vi "drive forward (1).vi"(8 "error in (no error)":errorcluster, 9 "forward":bool=TRUE, 10 "desired distance":dbl, 11 "RobotDriveDevRef in":T1) -> (0 "error out":errorcluster, 3 "RobotDriveDevRef out":T1)   [LabVIEW 2016]
uses:
  <vilib>/Rock Robotics/WPI/RobotDrive/WPI_RobotDriveDevRef.ctl
  <vilib>/Rock Robotics/WPI/MotorControl/WPI_MotorControlDeviceRef.ctl
  <vilib>/Rock Robotics/WPI/MotorControl/WPI_MotorControlType.ctl
  <vilib>/Rock Robotics/SystemInterfaces/DIO/FPGA_DIOPWMChannel.ctl
  <vilib>/Rock Robotics/WPI/PWM/WPI_PWMDeadband.ctl
  <vilib>/Rock Robotics/Network Tables/NT Write Number.vi
  <vilib>/Rock Robotics/WPI/RobotDrive/WPI_RobotDriveArcadeDrive_Standard(NoSaturation).vi
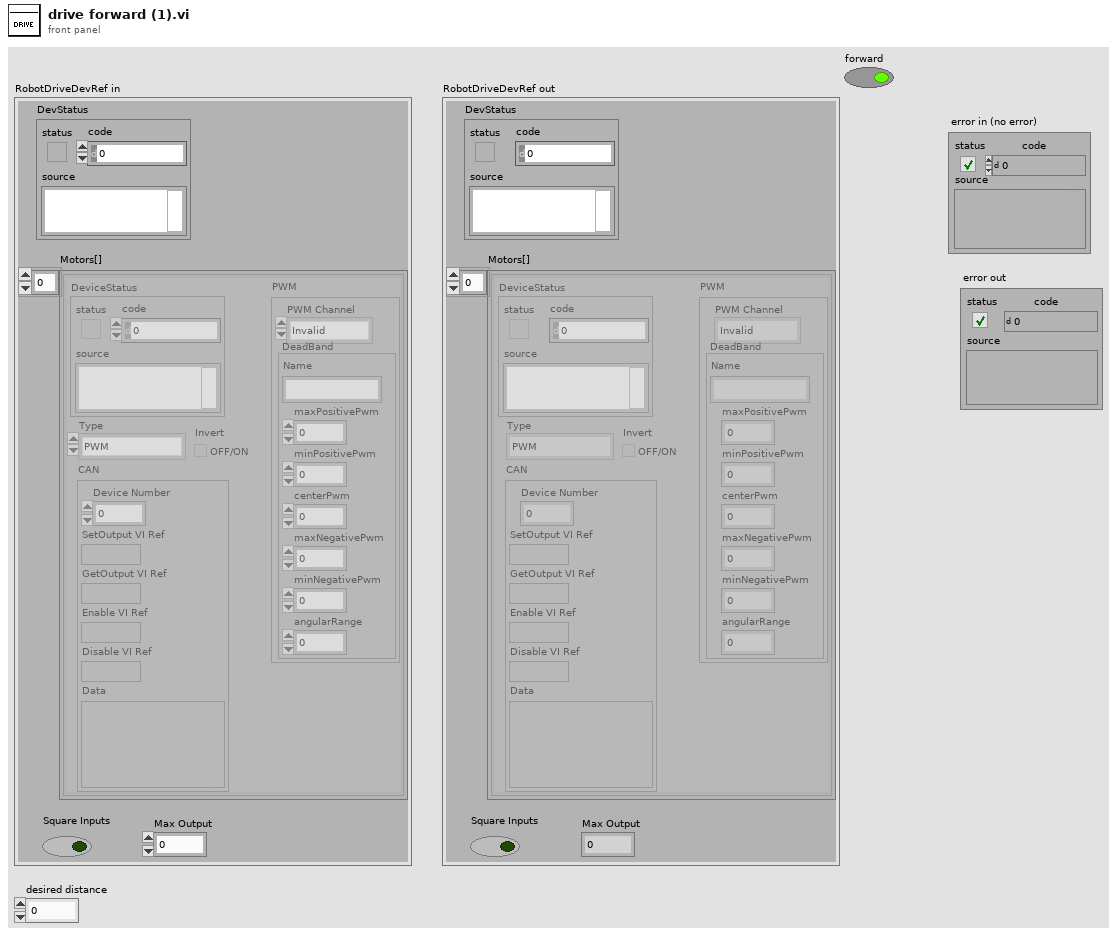
[diagram p1: front panel]
types:
  T1 = typedef "WPI_RobotDriveDevRef.ctl" = cluster{"DevStatus":errorcluster, "Motors[]":T2[], "Square Inputs":bool, "Max Output":dbl}
  T2 = typedef "WPI_MotorControlDeviceRef.ctl" = cluster{"DeviceStatus":errorcluster, "Type":T3, "PWM":cluster{"PWM Channel":T4, "DeadBand":T5}, "CAN":cluster{"Device Number":u8, "SetOutput VI Ref":variant, "GetOutput VI Ref":variant, "Enable VI Ref":variant, "Disable VI Ref":variant, "Data":variant}, "Invert":bool}
  T3 = typedef "WPI_MotorControlType.ctl" = enum16{"PWM", "CAN"}
  T4 = typedef "FPGA_DIOPWMChannel.ctl" = enum8{"PWM 0", "PWM 1", "PWM 2", "PWM 3", "PWM 4", "PWM 5", "PWM 6", "PWM 7", "PWM 8", "PWM 9", "PWM MXP 0", "PWM MXP 1", "PWM MXP 2", "PWM MXP 3", "PWM MXP 4", "PWM MXP 5", "PWM MXP 6", "PWM MXP 7", "PWM MXP 8", "PWM MXP 9", "Invalid"}
  T5 = typedef "WPI_PWMDeadband.ctl" = cluster{"Name":string, "maxPositivePwm":i32, "minPositivePwm":i32, "centerPwm":i32, "maxNegativePwm":i32, "minNegativePwm":i32, "angularRange":u16}
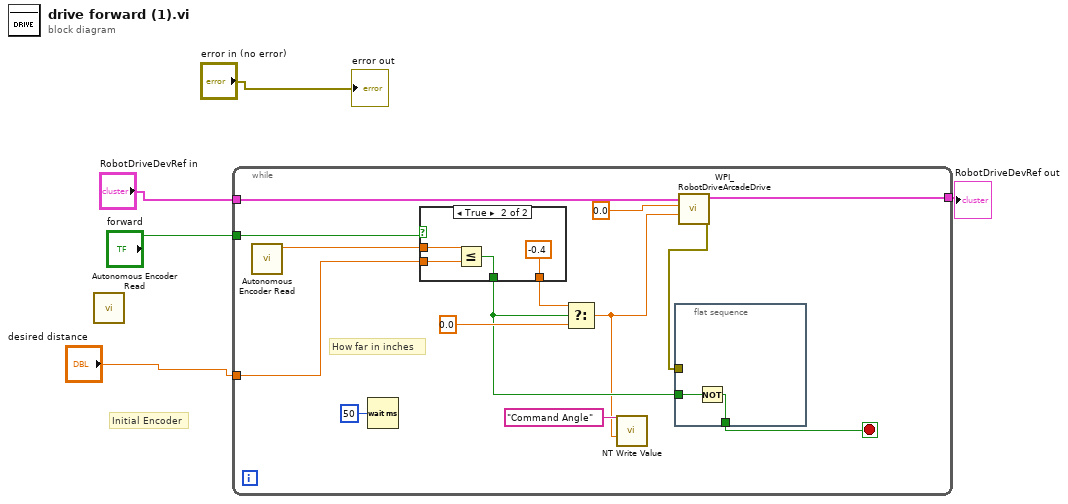
[diagram p0: block diagram]
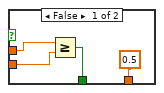
[diagram p2: hidden frame]
diagram:
  # "Initial Encoder"
  n1 = call "Autonomous Encoder Read.vi"() -> ()  [unwired: 9 in, 3 out]
  n2 = while {
    tunnel: "RobotDriveDevRef in" -> [w14]
    tunnel: [w13] -> w5
    tunnel: "desired distance" -> [w10]
    tunnel: "forward" -> [w8]
    stop <- w16 stop-if-true
    # "How far in inches"
    n3 = call "Autonomous Encoder Read.vi"() -> ("Encoder Distance"=w11:dbl)  [unwired: 9 in, 2 out]
    n4 = Wait (ms)(milliseconds to wait=u32 50) -> ()  [unwired: 1 out]
    n5 = case shown="True" w8 {
      tunnel: [0.5 ("t") -0.4 ("t")] -> w19
      tunnel: w11 -> [w21 w26]
      tunnel: w10 -> [w20 w25]
      tunnel: [w22 w24] -> w9
      frame False {
        n6 = Greater Or Equal?(x=w21, y=w20) -> (x >= y?=w22:bool)
      }
      frame True {
        n7 = Less Or Equal?(x=w26, y=w25) -> (x <= y?=w24:bool)
      }
    }
    n8 = Select(t=w19, s=w9, f=0.0) -> (s? t:f=w6:dbl)
    n9 = call-poly <vilib>:"NT Write Value.vi"("Numeric"=w6, "Name"="Command Angle") -> ()  [unwired: 9 in, 1 out]
    n10 = flat-sequence {
      tunnel: w9 -> [w29]
      tunnel: [w28] -> w16
      tunnel: w15 -> [_]
      frame #0 {
        n11 = Not(x=w29) -> (.not. x?=w28:bool)
      }
    }
    n12 = call-poly <vilib>:"WPI_RobotDriveArcadeDrive.vi"("Y axis value"=w6, "X axis value"=0.0, "RobotDriveDevRef"=w14) -> ("error out"=w15:errorcluster, "RobotDriveDevRef"=w13:T1)  [unwired: 6 in, 1 out]
  }
  "RobotDriveDevRef out" <- w5
  "error out" <- "error in (no error)"
